vi "Generate_I2C.vi"(8 "Error_In":errorcluster, 10 "Mode":T1, 11 "10Bit_Address_In":refnum<class "10 Bit Address.lvclass">) -> (0 "Error_Out":errorcluster, 3 "10Bit_Address_Out":refnum<class "10 Bit Address.lvclass">)   [LabVIEW 2021, in "10 Bit Address.lvclass"]
doc: "Used to generate the I2C Waveform for 10 bit register."
uses:
  10 Bit Address.lvclass
  Controls/I2C_States.ctl
  Controls/I2C_Data.ctl
  Controls/Customized_Ring.ctl
  Controls/Mode.ctl
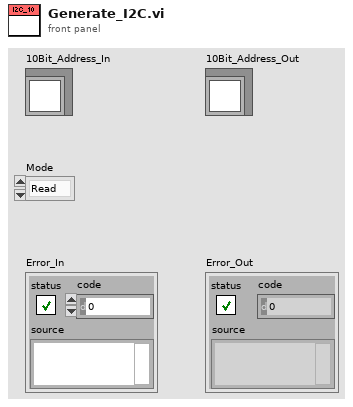
[diagram p1: front panel]
types:
  T1 = typedef "Mode.ctl" = enum16{"Read", "Write"}
  T2 = typedef "I2C_Data.ctl" = cluster{"Vmin":dbl, "Vmax":dbl, "Input":string, "Off_Set (uS)":dbl, "T_HD_STA (uS)":dbl, "Sample_Per_Us":dbl, "T_HD_DAT (uS)":dbl, "T_SU_DAT (uS)":dbl, "Frequency (kHz)":dbl, "T_SU_STO":dbl, "T_Off (uS)":dbl, "T_On (uS)":dbl, "T_BUF":dbl, "Target_Address":u16, "Selected_Register_Address":u8, "Byte_Array":u8[], "Target_Name":string, "Register_Name":string[], "Register_Address":u8[], "Target_Type":T3, "Register_Data":string[]}
  T3 = typedef "Customized_Ring.ctl" = u16
  T4 = typedef "I2C_States.ctl" = enum16{"Start", "Byte", "Ack_Nack", "Stop"}
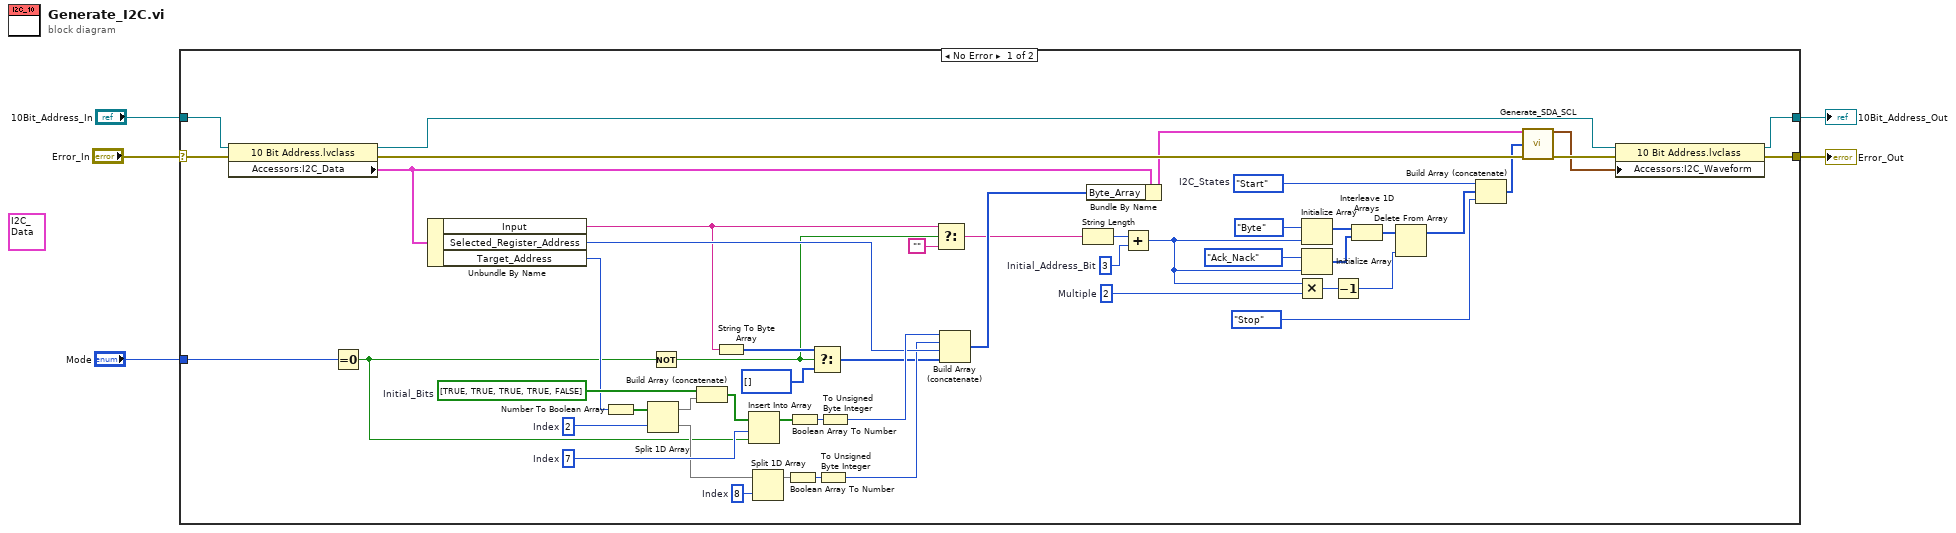
[diagram p0: block diagram]
diagram:
  (unwired) T2 {"Vmin"=0.0, "Vmax"=1.0, "Input"="", "Off_Set (uS)"=0.0, "T_HD_STA (uS)"=0.0, "Sample_Per_Us"=0.0, "T_HD_DAT (uS)"=0.0, "T_SU_DAT (uS)"=0.0, "Frequency (kHz)"=0.0, "T_SU_STO"=0.0, "T_Off (uS)"=0.0, "T_On (uS)"=0.0, "T_BUF"=0.0, "Target_Address"=0, "Selected_Register_Address"=0, "Byte_Array"=[], "Target_Name"="", "Register_Name"=[], "Register_Address"=[], "Target_Type"=0, "Register_Data"=[]} ("I2C_Data")
  n1 = case shown="No Error" "Error_In" {
    selector: "Error_In" -> [w55 w58]
    tunnel: [w33 w58] -> w1
    tunnel: [w35 w57] -> w2
    tunnel: "10Bit_Address_In" -> [w45 w57]
    tunnel: "Mode" -> [w42 _]
    frame No Error {
      w10 = 2  # Multiple
      w12 = 3  # Initial_Address_Bit
      w24 = 8  # Index
      w30 = bool[] [TRUE, TRUE, TRUE, TRUE, FALSE]  # Initial_Bits
      w31 = 2  # Index
      w41 = 7  # Index
      w53 = I2C_States."Start"  # I2C_States
      n2 = property on="Property Node" class="10 Bit Address.lvclass"(reference=w45, error in=w55) -> (reference out=w44:refnum<class "10 Bit Address.lvclass">, error out=w54:errorcluster, "Accessors:I2C_Data"=w34:T2)
      n3 = Equal To 0?(x=w42) -> (x = 0?=w17:bool)
      n4 = Unbundle By Name(w34) -> ("Input"=w8:string, "Selected_Register_Address"=w26:u8, "Target_Address"=w20:u16)
      n5 = Number To Boolean Array(number=w20) -> (Boolean array=w32:bool[])
      n6 = Split 1D Array(array=w32, index=w31) -> (first subarray=w29:bool[], second subarray=w25:bool[])
      n7 = Not(x=w17) -> (.not. x?=w9:bool)
      n8 = Build Array (concatenate)(w30, w29) -> (w28:bool[])
      n9 = String To Byte Array(string=w8) -> (unsigned byte array=w27:u8[])
      n10 = Insert Into Array(array=w28, index=w41, new element=w17) -> (w40:bool[])
      n11 = Split 1D Array(array=w25, index=w24) -> (first subarray=w22:bool[])  [unwired: 1 out]
      n12 = Boolean Array To Number(Boolean array=w22) -> (number=w23:u32)
      n13 = Boolean Array To Number(Boolean array=w40) -> (number=w39:u32)
      n14 = Select(t=w27, s=w9, f=u8[] []) -> (s? t:f=w19:u8[])
      n15 = To Unsigned Byte Integer(number=w23) -> (unsigned 8bit integer=w21:u8)
      n16 = To Unsigned Byte Integer(number=w39) -> (unsigned 8bit integer=w38:u8)
      n17 = Select(t=w8, s=w9, f="") -> (s? t:f=w7:string)
      n18 = Build Array (concatenate)(w38, w21, w26, w19) -> (w36:u8[])
      n19 = String Length(string=w7) -> (length=w51:i32)
      n20 = Bundle By Name(cluster=w34, "Byte_Array"=w36) -> (w37:T2)
      n21 = Add(x=w51, y=w12) -> (x+y=w13:i32)
      n22 = Multiply(x=w13, y=w10) -> (x*y=w16:i32)
      n23 = Initialize Array(I2C_States."Byte" ("Enum"), w13) -> (w49:T4[])
      n24 = Initialize Array(I2C_States."Ack_Nack" ("element"), w13) -> (w48:T4[])
      n25 = Decrement(x=w16) -> (x-1=w15:i32)
      n26 = Interleave 1D Arrays(w49, w48) -> (w14:T4[])
      n27 = Delete From Array(array=w14, index=w15) -> (array with subset deleted=w11:T4[])  [unwired: 1 in, 1 out]
      n28 = Build Array (concatenate)(w53, w11, I2C_States."Stop" ("element")) -> (w46:T4[])
      n29 = call "Generate_SDA_SCL.vi"("Data"=w37, "Data_Sequence"=w46, "Error_In"=w54) -> ("Waveform Graph"=w43:waveform(dbl)[], "Error_Out"=w56:errorcluster)  [unwired: 11 in]
      n30 = property class="10 Bit Address.lvclass"(reference=w44, error in=w56, "Accessors:I2C_Waveform"=w43) -> (reference out=w35:refnum<class "10 Bit Address.lvclass">, error out=w33:errorcluster)
    }
    frame Error {
    }
  }
  "Error_Out" <- w1
  "10Bit_Address_Out" <- w2
